vi "Test Results Are Not Added to All Test Cases beginning with Name.vi"(8 "error in (no error)":errorcluster, 11 "Result Model Result Recording Test in":refnum<class "Result Model Result Recording Test.lvclass">) -> (0 "error out":errorcluster, 3 "Result Model Result Recording Test out":refnum<class "Result Model Result Recording Test.lvclass">)   [LabVIEW 2020, in "Result Model Result Recording Test.lvclass"]
uses:
  Result Model Result Recording Test.lvclass
  source/Core/Result/Type.ctl
  source/Core/Result/Result.lvlib
  source/Core/Result/Status.ctl
  source/Core/Result/Result.ctl
  source/User Interface/Result Model by Reference/Result Model by Reference.lvclass
  ae2c71b8-32bb-49d1-8500-0119bfec74ff.vi
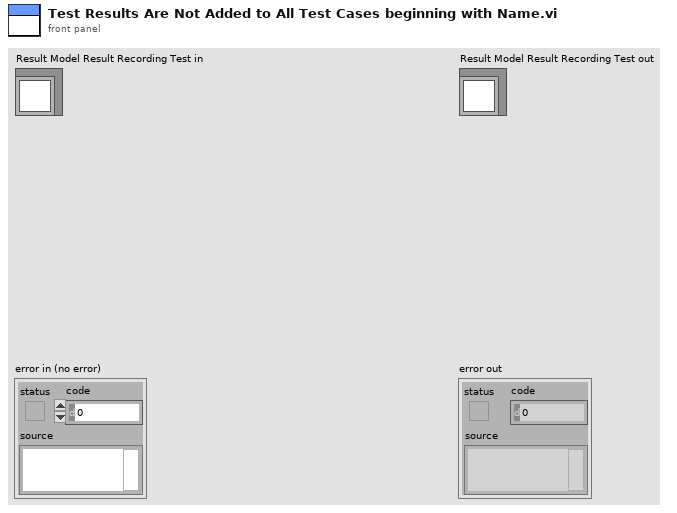
[diagram p1: front panel]
types:
  T1 = typedef "Result.lvlib/Result.ctl" = cluster{"Name":string, "Description":string, "Status":T2, "Result Type":T3, "Execution Time":dbl, "Data":cluster{"Expected":variant, "Actual":variant, "Delta":variant}}
  T2 = typedef "Result.lvlib/Status.ctl" = enum16{"", "Passed", "Failed", "Error", "Skipped", "Setup Error", "Broken", "Teardown Error"}
  T3 = typedef "Result.lvlib/Type.ctl" = enum16{"Test Case", "Test Suite", "Test Run", "Pass", "Fail", "Skip", "Pass if", "Fail if", "Pass if Error", "Fail if Error", "Pass if Equal", "Fail if Equal"}
  T4 = cluster{"Left Cell String":string, "Child Text":string[], "Child Tag":string, "Item Indent":i32, "Child Only?":bool, "Glyph Index":i32}[]
  T5 = cluster{"Left Cell String":string, "Child Text":string[], "Child Tag":string, "Item Indent":i32, "Child Only?":bool, "Glyph Index":i32}
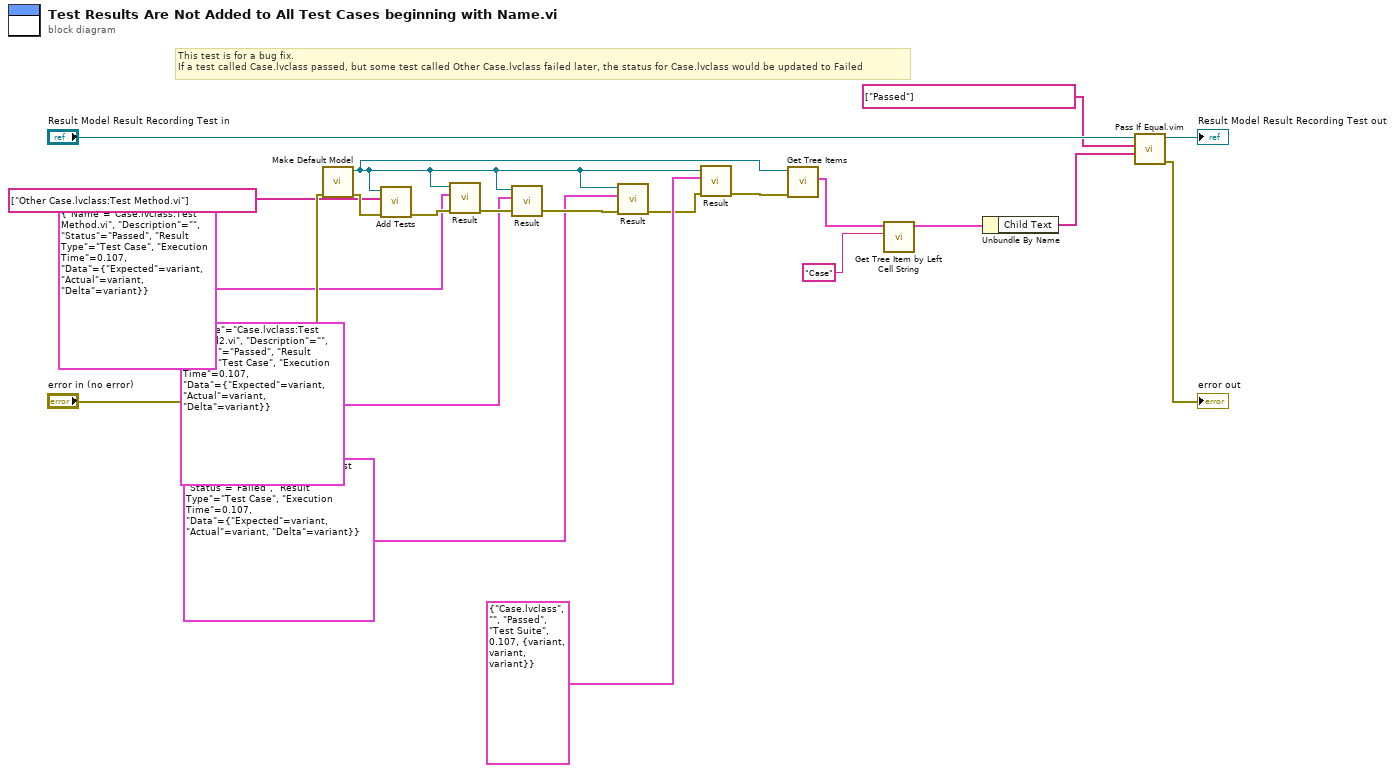
[diagram p0: block diagram]
diagram:
  # "This test is for a bug fix. \nIf a test called Case.lvclass passed, but some test called Other Case.lvclass failed later, the status for Case.lvclass would be updated to Failed"
  n1 = call "Make Default Model.vi"("error in (no error)"="error in (no error)") -> ("error out"=w9:errorcluster, "Result Model out"=w3:refnum<class "Result Model by Reference.lvclass">)  [unwired: 9 in]
  n2 = call "Add Tests.vi"("error in (no error)"=w9, "Tests"=string[] ["Other Case.lvclass:Test Method.vi"] ("String"), "Result Model by Reference In"=w3) -> ("error out"=w7:errorcluster)  [unwired: 8 in]
  n3 = call-dynamic "Result.vi"("error in (no error)"=w7, "Results"=T1 {"Name"="Case.lvclass:Test Method.vi", "Description"="", "Status"=enum."Passed", "Result Type"=enum."Test Case", "Execution Time"=0.107, "Data"={"Expected"=variant, "Actual"=variant, "Delta"=variant}} ("Result"), "Result Model by Reference In"=w3) -> ("error out"=w5:errorcluster)  [unwired: 8 in]
  n4 = call-dynamic "Result.vi"("Results"=T1 {"Name"="Case.lvclass:Test Method2.vi", "Description"="", "Status"=enum."Passed", "Result Type"=enum."Test Case", "Execution Time"=0.107, "Data"={"Expected"=variant, "Actual"=variant, "Delta"=variant}} ("Result"), "Result Model by Reference In"=w3) -> ()  [unwired: 9 in, 1 out]
  n5 = call-dynamic "Result.vi"("error in (no error)"=w5, "Results"=T1 {"Name"="Other Case.lvclass:Test Method.vi", "Description"="", "Status"=enum."Failed", "Result Type"=enum."Test Case", "Execution Time"=0.107, "Data"={"Expected"=variant, "Actual"=variant, "Delta"=variant}} ("Result"), "Result Model by Reference In"=w3) -> ("error out"=w4:errorcluster)  [unwired: 8 in]
  n6 = call-dynamic "Result.vi"("error in (no error)"=w4, "Results"=T1 {"Name"="Case.lvclass", "Description"="", "Status"=enum."Passed", "Result Type"=enum."Test Suite", "Execution Time"=0.107, "Data"={"Expected"=variant, "Actual"=variant, "Delta"=variant}} ("Result"), "Result Model by Reference In"=w3) -> ("error out"=w10:errorcluster)  [unwired: 8 in]
  n7 = call "Get Tree Items.vi"("error in (no error)"=w10, "Result Model by Reference In"=w3) -> ("Tree Items"=w20:T4)  [unwired: 8 in, 1 out]
  n8 = call "Get Tree Item by Left Cell String.vi"("Left Cell String"="Case", "Tree Items"=w20) -> ("Item"=w16:T5)  [unwired: 9 in]
  n9 = Unbundle By Name(w16) -> ("Child Text"=w15:string[])
  n10 = call "Pass If Equal.vim"("Actual"=w15, "Expected"=string[] ["Passed"] ("Child Text"), "LUnit Test Case In"="Result Model Result Recording Test in") -> ("error out"=→"error out":errorcluster, "LUnit Test Case Out"=→"Result Model Result Recording Test out":refnum<class "Result Model Result Recording Test.lvclass">)  [unwired: 7 in]
